vi "MM6.DetermineRepetitionPattern.vi"(11 "string":string) -> (2 "MatchPattern":T1, 3 "string out":string)   [LabVIEW 2014, in "MM6.lvlib"]
doc: "This vi determines the repetition pattern.\n\nauthor: Christopher Borgmann, christopher.borgmann@cern.ch"
uses:
  MM6.lvlib
  MM6.MatchRepPattern.ctl
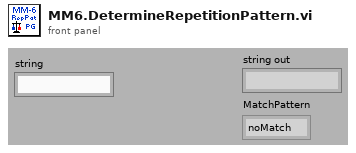
[diagram p1: front panel]
types:
  T1 = typedef "MM6.lvlib/MM6.MatchRepPattern.ctl" = enum16{"noMatch", "oneTG", "twoTG"}
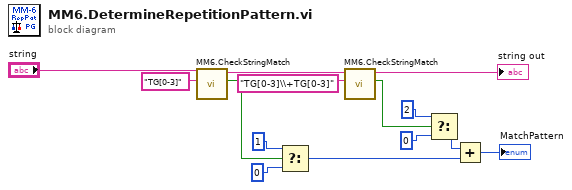
[diagram p0: block diagram]
diagram:
  n1 = call "MM6.CheckStringMatch.vi"("regular expression"="TG[0-3]", "string"="string") -> ("exact match?"=w10:bool, "string out"=w12:string)  [unwired: 8 in]
  n2 = Select(t=u16 1, s=w10, f=u16 0) -> (s? t:f=w3:u16)
  n3 = call "MM6.CheckStringMatch.vi"("regular expression"="TG[0-3]\\+TG[0-3]", "string"=w12) -> ("exact match?"=w5:bool, "string out"=→"string out":string)  [unwired: 8 in]
  n4 = Select(t=u16 2, s=w5, f=u16 0) -> (s? t:f=w4:u16)
  n5 = Add(x=w4, y=w3) -> (x+y=→"MatchPattern":u16)
